vi "Configure Basic Level Measurement.vi"(7 "Append Traces (T: Enable)":bool=TRUE, 8 "error in (no error)":errorcluster, 9 "Selection Type (0: mLevel)":i32(ring) items=["mLevel", "mRatio"], 10 "Waveform (0: wsSine)":i32(ring) items=["wsSine", "wsLDSine"], 11 "VISA resource name":refnum<visa-resource-name>) -> (0 "error out":errorcluster, 3 "VISA resource name out":refnum<visa-resource-name>)   [LabVIEW 2014, in "Stanford Research SR1.lvlib"]
doc: "Configures the basic attributes for the Level Quick Measurement."
uses:
  Stanford Research SR1.lvlib
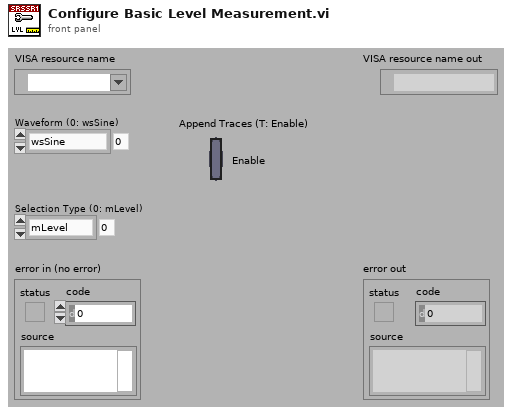
[diagram p1: front panel]
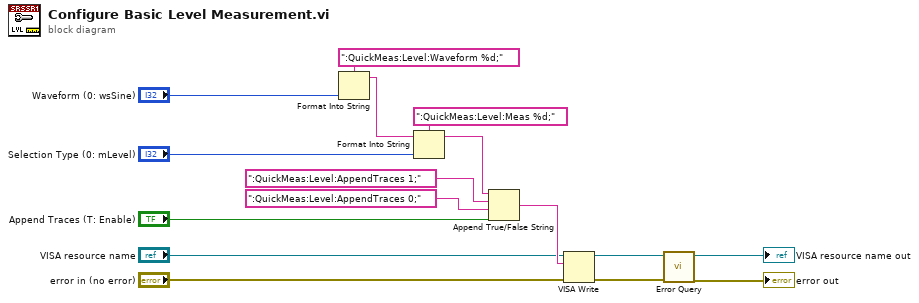
[diagram p0: block diagram]
diagram:
  n1 = Format Into String(format string=":QuickMeas:Level:Waveform %d;", "Waveform (0: wsSine)") -> (resulting string=w14:string)  [unwired: 2 in, 1 out]
  n2 = Format Into String(format string=":QuickMeas:Level:Meas %d;", initial string=w14, "Selection Type (0: mLevel)") -> (resulting string=w11:string)  [unwired: 1 in, 1 out]
  n3 = Append True/False String(1:"Append Traces (T: Enable)", 2:":QuickMeas:Level:AppendTraces 0;", 3:":QuickMeas:Level:AppendTraces 1;", 4:w11) -> (0:w7:string)
  n4 = VISA Write(VISA resource name="VISA resource name", write buffer=w7, error in (no error)="error in (no error)") -> (VISA resource name out=w4:refnum<visa-resource-name>, error out=w3:errorcluster)  [unwired: 1 out]
  n5 = call "Error Query.vi"("error in (no error)"=w3, "VISA resource name"=w4) -> ("error out"=→"error out":errorcluster, "VISA resource name out"=→"VISA resource name out":refnum<visa-resource-name>)  [unwired: 6 in, 2 out]
